vi "Pressure Launcher.vi"(9 "Sub Panel":refnum<vi>, 10 "Sensor ID":enum16{"Chamber", "Feeder"}(ring), 11 "Panel Actor In":refnum<class "Main.lvclass">) -> (2 "Nested Actor's Enqueuer":refnum<class "Message Enqueuer.lvclass">, 3 "Panel Actor Out":refnum<class "Main.lvclass">)   [LabVIEW 2018, in "Pressure Actor.lvlib" / "Pressure.lvclass"]
uses:
  Pressure.lvclass
  <vilib>/ActorFramework/Message Enqueuer/Message Enqueuer.lvclass
  ADM/ADM/Main.lvclass
  C:/Program Files (x86)/National Instruments/LabVIEW 2018/vi.lib/MGI/Panel Manager/Panel Actor/Panel Actor/Panel Actor.lvclass
  Pressure.lvclass/Pressure.ctl
  <vilib>/MGI/Panel Manager/Panel/Panel/Subpanel/Subpanel.lvclass
  C:/Program Files (x86)/National Instruments/LabVIEW 2018/vi.lib/MGI/Panel Manager/Panel/Panel/Panel.lvclass
  <vilib>/MGI/Panel Manager/Panel/Panel/Subpanel/Subpanel.vi
  <vilib>/MGI/Panel Manager/Panel/Panel.lvlib
  <vilib>/MGI/Panel Manager/Panel Actor/Panel Actor/Panel Actor.lvclass
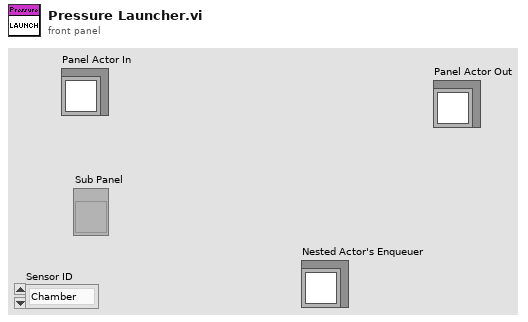
[diagram p1: front panel]
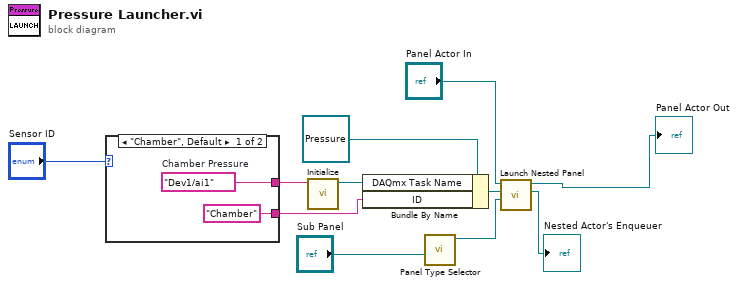
[diagram p0: block diagram]
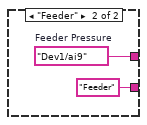
[diagram p2: hidden frame]
diagram:
  n1 = case shown="\"Chamber\", Default" "Sensor ID" {
    tunnel: [w13 w15] -> w4
    tunnel: ["Chamber" ("ID") "Feeder" ("ID")] -> w3
    frame "Chamber", Default {
      w13 = tag "Dev1/ai1"  # Chamber Pressure
    }
    frame "Feeder" {
      w15 = tag "Dev1/ai9"  # Feeder Pressure
    }
  }
  n2 = call "Initialize.vi"("physical channels"=w4) -> ("task out"=w2:refnum<k21>)  [unwired: 9 in, 1 out]
  n3 = Bundle By Name(cluster=refnum<class "Pressure.lvclass"> refnum ("Pressure Actor.lvlib:Pressure.lvclass"), "DAQmx Task Name"=w2, "ID"=w3) -> (w5:refnum<class "Pressure.lvclass">)
  n4 = call-poly <vilib>:"Panel Type Selector.vi"("Sub Panel"="Sub Panel") -> ("Subpanel Out"=w9:refnum<class "Subpanel.lvclass">)  [unwired: 9 in, 1 out]
  n5 = call <vilib>:"Launch Nested Panel.vi"("Panel"=w9, "Nested Panel Actor"=w5, "Panel Actor in"="Panel Actor In") -> ("Nested Actor's Enqueuer"=→"Nested Actor's Enqueuer":refnum<class "Message Enqueuer.lvclass">, "Panel Actor out"=→"Panel Actor Out":refnum<class "Main.lvclass">)  [unwired: 5 in, 2 out]
